vi "Start.vi"() -> ()   [LabVIEW 2017]
uses:
  <vilib>/Utility/config.llb/NI_LVConfig.lvlib
panel:
  out "Automation":bool
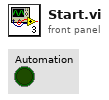
[diagram p1: front panel]
types:
  T1 = enum16{"End", "Start", "Verify VR", "Verify UUT"}
  T2 = enum16{"Auxiliary", "Temp Sens Cal", "Com Test", "Enable Test", "Speed Command", "Stop Time", "Temp Control", "Burn in", "Visual Inspec", "Empty"}
  T3 = enum16{"Auxiliary", "Temp Sens Cal", "Com Test", "Enable Test", "Speed Command", "Stop Time", "Temp Control", "Burn in", "Visual Inspec", "Empty"}[]
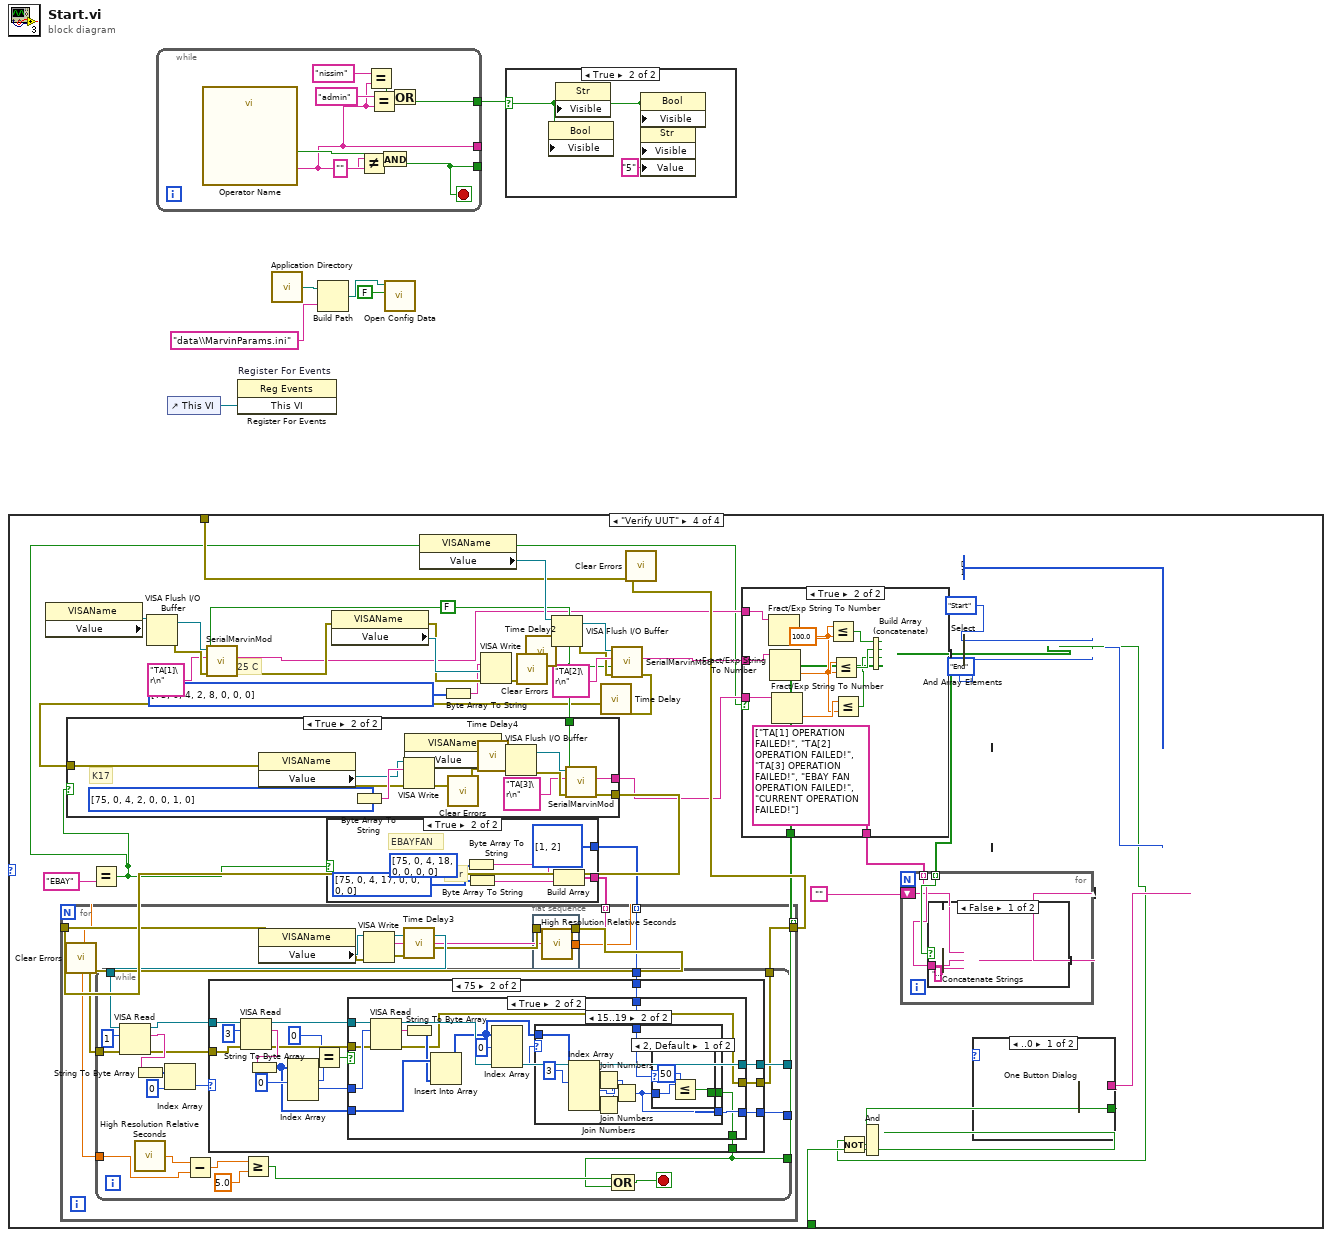
[diagram p0: block diagram]
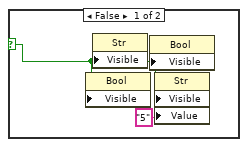
[diagram p2: hidden frame]
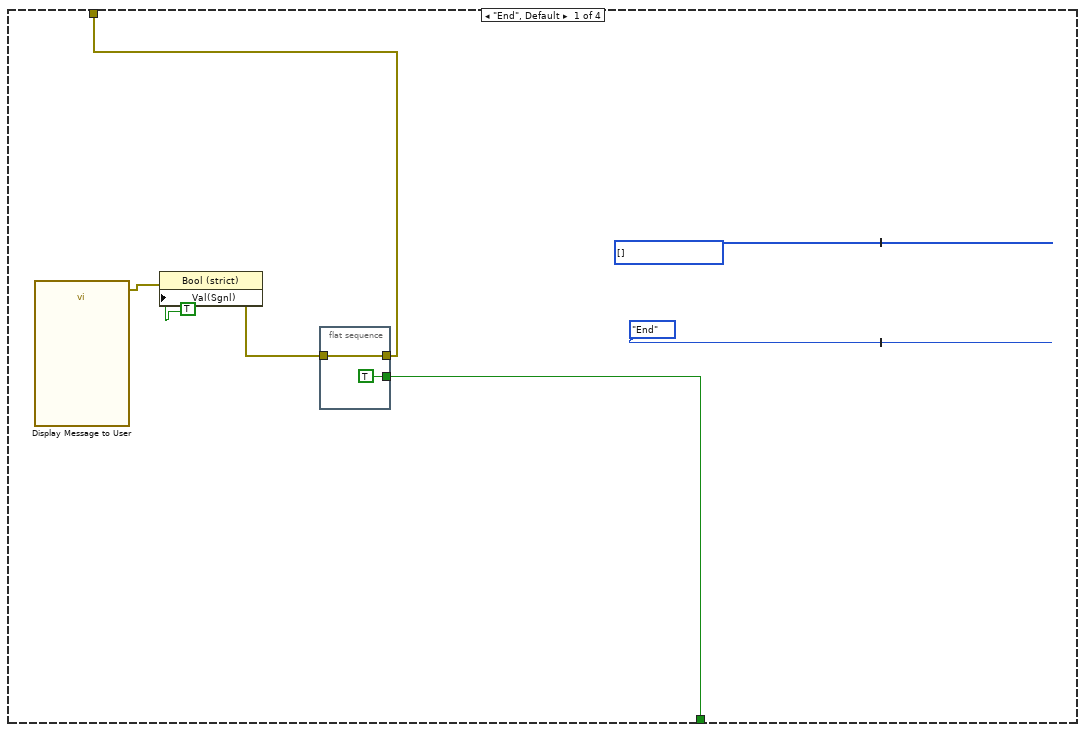
[diagram p3: hidden frame]
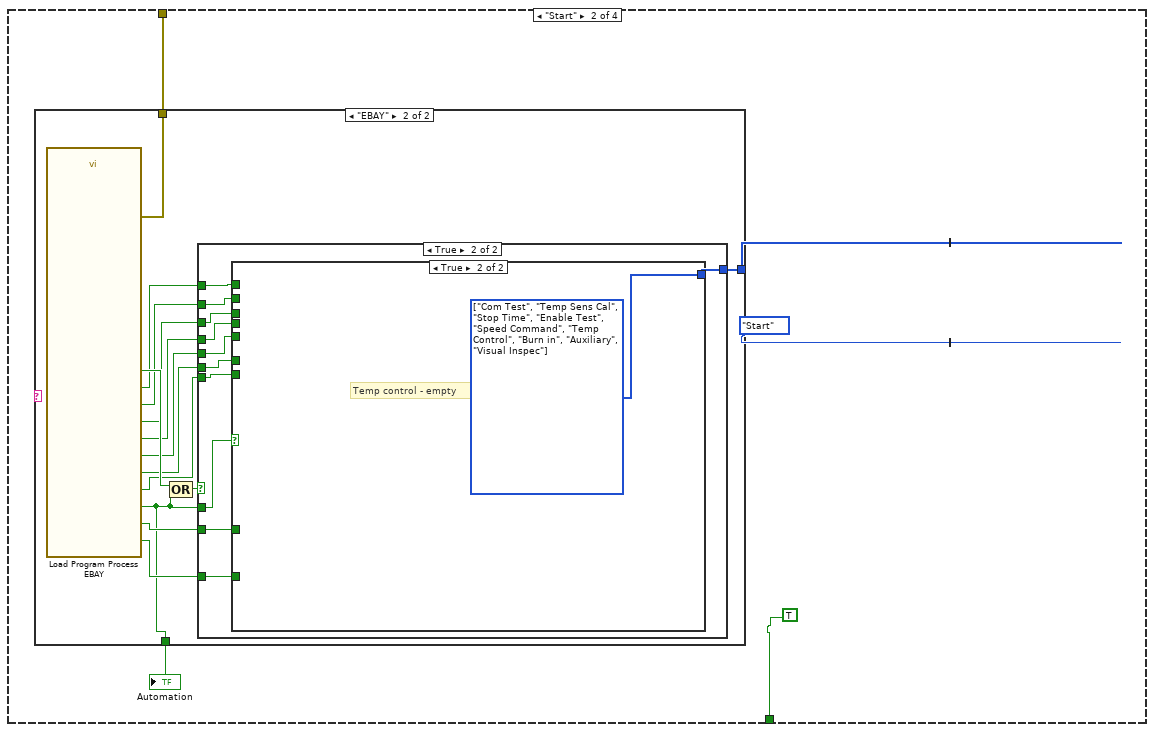
[diagram p4: hidden frame]
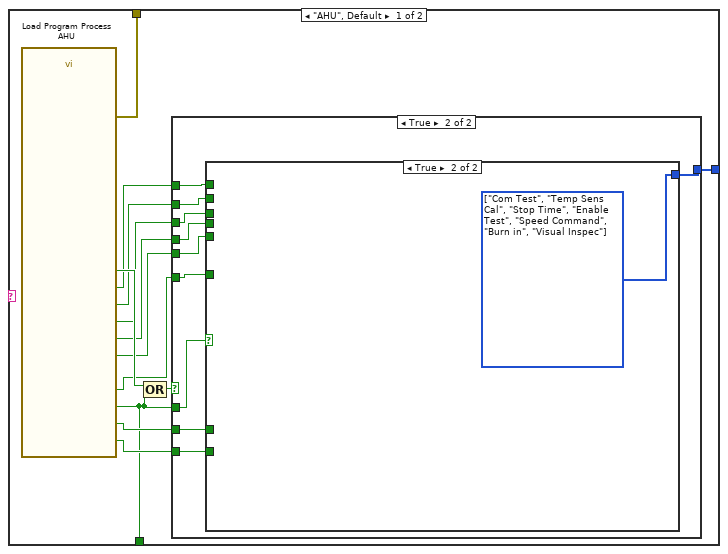
[diagram p5: hidden frame]
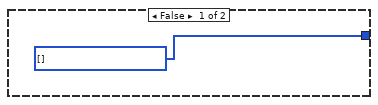
[diagram p6: hidden frame]
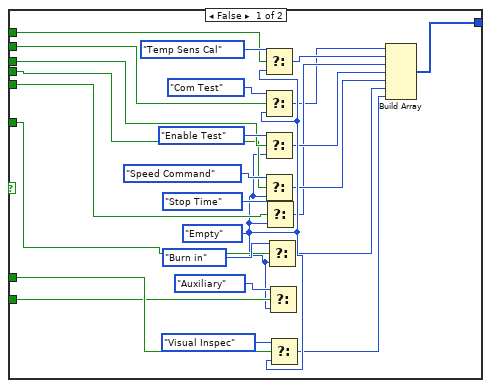
[diagram p7: hidden frame]
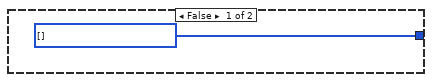
[diagram p8: hidden frame]
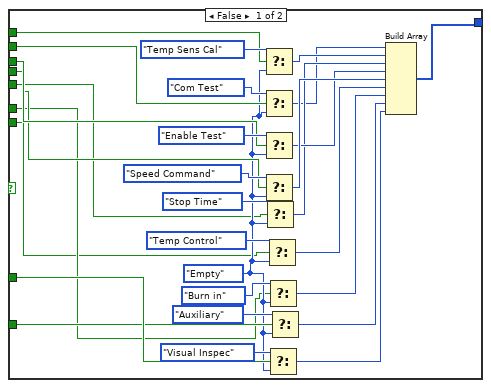
[diagram p9: hidden frame]
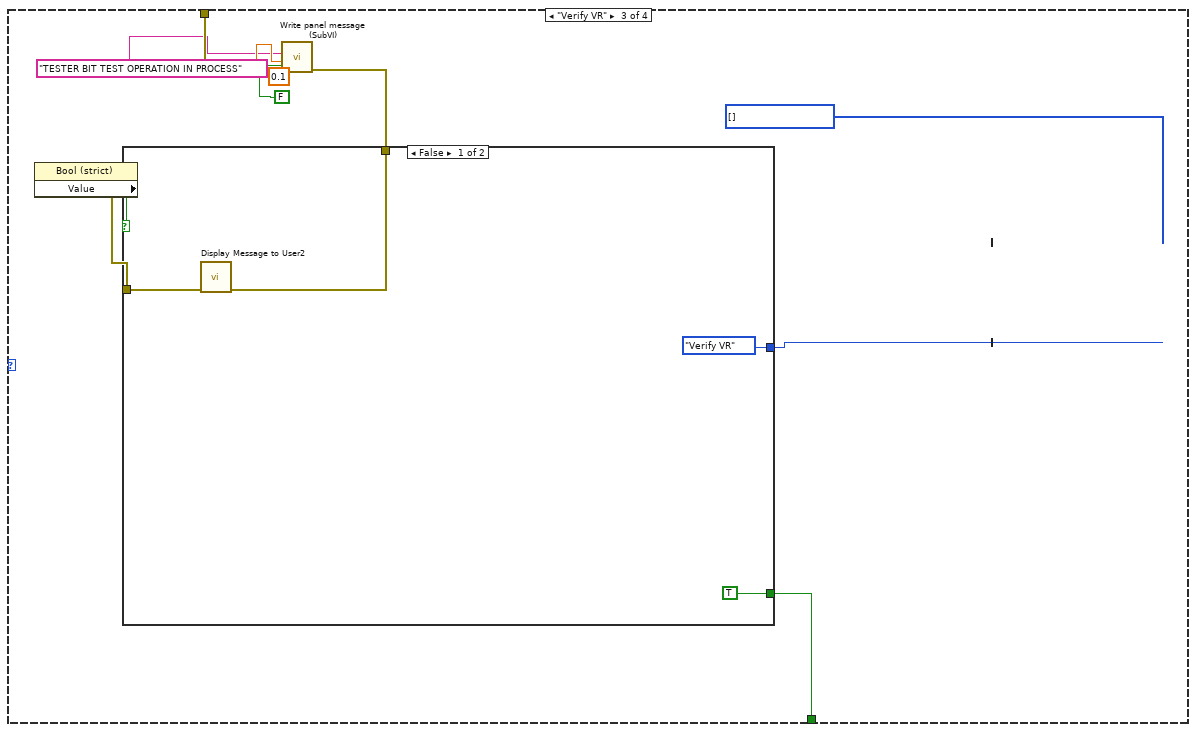
[diagram p10: hidden frame]
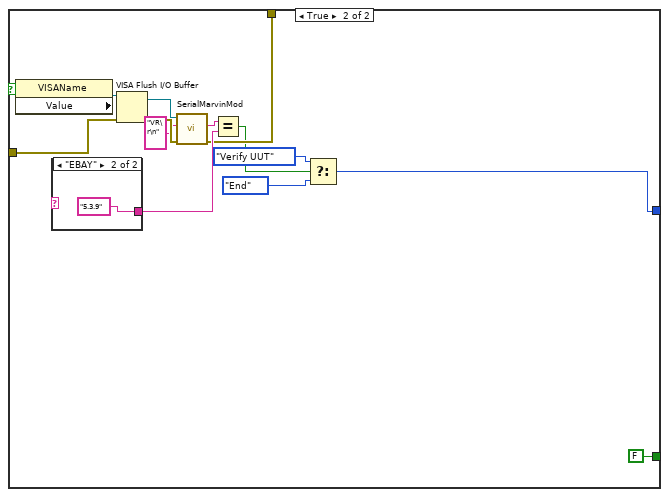
[diagram p11: hidden frame]
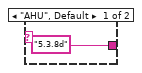
[diagram p12: hidden frame]
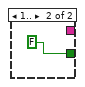
[diagram p13: hidden frame]
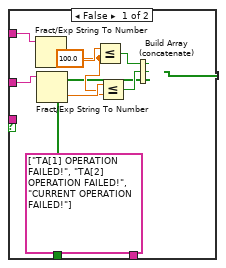
[diagram p14: hidden frame]
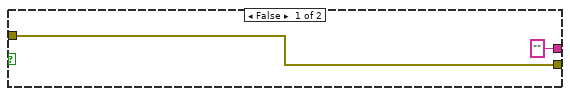
[diagram p15: hidden frame]
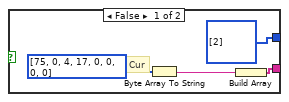
[diagram p16: hidden frame]
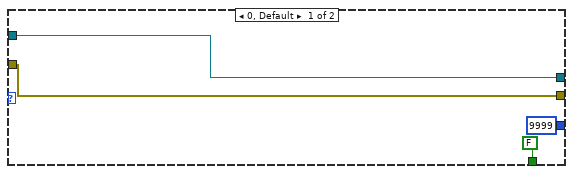
[diagram p17: hidden frame]
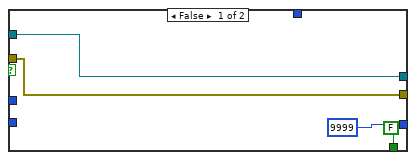
[diagram p18: hidden frame]
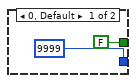
[diagram p19: hidden frame]
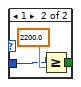
[diagram p20: hidden frame]
diagram:
  n1 = case shown="\"Verify UUT\"" {
    selector: _ -> [_ _ _ _]
    tunnel: [w10 w20 w130 w178] -> _
    tunnel: [w12 w19 w135 w156] -> _
    tunnel: [T1."End" T1."Start" w136 w172] -> _
    tunnel: [w11 TRUE w131 w166] -> _
    frame "End", Default {
      w12 = T3 [] items=["Auxiliary", "Temp Sens Cal", "Com Test", "Enable Test", "Speed Command", "Stop Time", "Temp Control", "Burn in", "Visual Inspec", "Empty"]
      n2 = call "Display Message to User"() -> ("error out"=w7:errorcluster)  [unwired: 10 in, 1 out]
      n3 = property on="Property Node" class="Bool (strict)"(error in=w7, "Val(Sgnl)"=TRUE ("Value (Signaling)")) -> (error out=w8:errorcluster)  [unwired: 1 in, 1 out]
      n4 = flat-sequence {
        tunnel: w8 -> [w14]
        tunnel: [TRUE] -> w11
        tunnel: [w14] -> w10
        frame #0 {
        }
      }
    }
    frame "Start" {
      n5 = case shown="\"EBAY\"" {
        selector: _ -> [_ _]
        tunnel: [w33 w84] -> w19
        tunnel: [w32 w83] -> w20
        tunnel: [w21 w71] -> w16
        frame "AHU", Default {
          n6 = call "Load Program Process AHU.vi"() -> ("Speed Command Test"=w26:bool, "Enable Test"=w27:bool, "Burn-in Test"=w24:bool, "Auxiliary"=w22:bool, "Temperature Sensor Calibration Test"=w29:bool, "Communication Test"=w28:bool, "Motor Temperature Test"=w25:bool, "Visual Inspection"=w23:bool, "OK"=w30:bool, "Automation"=w21:bool, "error out"=w32:errorcluster)  [unwired: 8 in, 9 out]
          n7 = Compound Arithmetic op=OR(w30, w21) -> (w31:bool)
          n8 = case shown="True" w31 {
            tunnel: [w34 w44] -> w33
            tunnel: w21 -> [_ w43]
            tunnel: w29 -> [_ w42]
            tunnel: w28 -> [_ w41]
            tunnel: w27 -> [_ w40]
            tunnel: w26 -> [_ w39]
            tunnel: w25 -> [_ w38]
            tunnel: w24 -> [_ w37]
            tunnel: w23 -> [_ w36]
            tunnel: w22 -> [_ w35]
            frame False {
              w34 = T3 [] items=["Auxiliary", "Temp Sens Cal", "Com Test", "Enable Test", "Speed Command", "Stop Time", "Temp Control", "Burn in", "Visual Inspec", "Empty"]
            }
            frame True {
              n9 = case shown="True" w43 {
                tunnel: [w69 w70] -> w44
                tunnel: w42 -> [w61 _]
                tunnel: w41 -> [w60 _]
                tunnel: w40 -> [w59 _]
                tunnel: w39 -> [w58 _]
                tunnel: w38 -> [w57 _]
                tunnel: w37 -> [w56 _]
                tunnel: w36 -> [w55 _]
                tunnel: w35 -> [w54 _]
                frame False {
                  w52 = T2."Empty" ("f")
                  n10 = Select(t=T2."Temp Sens Cal" ("f"), s=w61, f=w52) -> (s? t:f=w46:T2)
                  n11 = Select(t=T2."Com Test" ("f"), s=w60, f=w52) -> (s? t:f=w45:T2)
                  n12 = Select(t=T2."Enable Test" ("f"), s=w59, f=w52) -> (s? t:f=w48:T2)
                  n13 = Select(t=T2."Speed Command" ("f"), s=w58, f=w52) -> (s? t:f=w49:T2)
                  n14 = Select(t=T2."Stop Time" ("f"), s=w57, f=w52) -> (s? t:f=w47:T2)
                  n15 = Select(t=T2."Burn in" ("f"), s=w56, f=w52) -> (s? t:f=w50:T2)
                  n16 = Select(t=T2."Auxiliary" ("f"), s=w54, f=w52) -> ()  [unwired: 1 out]
                  n17 = Select(t=T2."Visual Inspec" ("f"), s=w55, f=w52) -> (s? t:f=w51:T2)
                  n18 = Build Array(w45, w46, w47, w48, w49, w50, w51) -> (w69:T3)
                }
                frame True {
                  w70 = T3 [enum."Com Test", enum."Temp Sens Cal", enum."Stop Time", enum."Enable Test", enum."Speed Command", enum."Burn in", enum."Visual Inspec"] items=["Auxiliary", "Temp Sens Cal", "Com Test", "Enable Test", "Speed Command", "Stop Time", "Temp Control", "Burn in", "Visual Inspec", "Empty"]
                }
              }
            }
          }
        }
        frame "EBAY" {
          n19 = call "Load Program Process EBAY.vi"() -> ("Speed Command Test"=w77:bool, "Enable Test"=w78:bool, "Burn-in Test"=w75:bool, "Temperature Control Algorithm Test"=w74:bool, "Auxiliary"=w72:bool, "Temperature Sensor Calibration Test"=w80:bool, "Communication Test"=w79:bool, "Motor Temperature Test"=w76:bool, "Visual Inspection"=w73:bool, "OK"=w81:bool, "Automation"=w71:bool, "error out"=w83:errorcluster)  [unwired: 8 in, 8 out]
          n20 = Compound Arithmetic op=OR(w81, w71) -> (w82:bool)
          n21 = case shown="True" w82 {
            tunnel: [w85 w96] -> w84
            tunnel: w71 -> [_ w95]
            tunnel: w80 -> [_ w94]
            tunnel: w79 -> [_ w93]
            tunnel: w78 -> [_ w92]
            tunnel: w77 -> [_ w91]
            tunnel: w76 -> [_ w90]
            tunnel: w75 -> [_ w89]
            tunnel: w74 -> [_ w88]
            tunnel: w73 -> [_ w87]
            tunnel: w72 -> [_ w86]
            frame False {
              w85 = T3 [] items=["Auxiliary", "Temp Sens Cal", "Com Test", "Enable Test", "Speed Command", "Stop Time", "Temp Control", "Burn in", "Visual Inspec", "Empty"]
            }
            frame True {
              n22 = case shown="True" w95 {
                tunnel: [w125 w126] -> w96
                tunnel: w94 -> [w116 _]
                tunnel: w93 -> [w115 _]
                tunnel: w92 -> [w114 _]
                tunnel: w91 -> [w113 _]
                tunnel: w90 -> [w103 _]
                tunnel: w89 -> [w108 _]
                tunnel: w88 -> [w107 _]
                tunnel: w87 -> [w112 _]
                tunnel: w86 -> [w111 _]
                frame False {
                  w109 = T2."Empty" ("f")
                  n23 = Select(t=T2."Temp Sens Cal" ("f"), s=w116, f=w109) -> (s? t:f=w98:T2)
                  n24 = Select(t=T2."Com Test" ("f"), s=w115, f=w109) -> (s? t:f=w97:T2)
                  n25 = Select(t=T2."Enable Test" ("f"), s=w114, f=w109) -> (s? t:f=w100:T2)
                  n26 = Select(t=T2."Speed Command" ("f"), s=w113, f=w109) -> (s? t:f=w101:T2)
                  n27 = Select(t=T2."Stop Time" ("f"), s=w103, f=w109) -> (s? t:f=w99:T2)
                  n28 = Select(t=T2."Temp Control" ("f"), s=w107, f=w109) -> (s? t:f=w102:T2)
                  n29 = Select(t=T2."Burn in" ("f"), s=w108, f=w109) -> (s? t:f=w104:T2)
                  n30 = Select(t=T2."Visual Inspec" ("f"), s=w112, f=w109) -> (s? t:f=w106:T2)
                  n31 = Select(t=T2."Auxiliary" ("f"), s=w111, f=w109) -> (s? t:f=w105:T2)
                  n32 = Build Array(w97, w98, w99, w100, w101, w102, w104, w105, w106) -> (w125:T3)
                }
                frame True {
                  w126 = T3 [enum."Com Test", enum."Temp Sens Cal", enum."Stop Time", enum."Enable Test", enum."Speed Command", enum."Temp Control", enum."Burn in", enum."Auxiliary", enum."Visual Inspec"] items=["Auxiliary", "Temp Sens Cal", "Com Test", "Enable Test", "Speed Command", "Stop Time", "Temp Control", "Burn in", "Visual Inspec", "Empty"]
                  # "Temp control - empty"
                }
              }
            }
          }
        }
      }
      "Automation" <- w16
    }
    frame "Verify VR" {
      w135 = T3 [] items=["Auxiliary", "Temp Sens Cal", "Com Test", "Enable Test", "Speed Command", "Stop Time", "Temp Control", "Burn in", "Visual Inspec", "Empty"]
      n33 = property on="Property Node" class="Bool (strict)"() -> (error out=w133:errorcluster, "Value"=w132:bool)  [unwired: 2 in, 1 out]
      n34 = case shown="False" w132 {
        tunnel: w133 -> [w140 w149]
        tunnel: [T1."Verify VR" w144] -> w136
        tunnel: [w138 w143] -> w134
        tunnel: [TRUE FALSE] -> w131
        frame False {
          n35 = call "Display Message to User2"("error in (no error)"=w140) -> ("error out"=w138:errorcluster)  [unwired: 9 in, 1 out]
        }
        frame True {
          n36 = property on="Property Node" class="VISAName"() -> ("Value"=w151:refnum<visa-resource-name>)  [unwired: 2 in, 2 out]
          n37 = case shown="\"EBAY\"" {
            selector: _ -> [_ _]
            tunnel: ["5.3.8d" ("write buffer") "5.3.9" ("write buffer")] -> w147
            frame "AHU", Default {
            }
            frame "EBAY" {
            }
          }
          n38 = VISA Flush I/O Buffer(VISA resource name=w151, error in (no error)=w149) -> (VISA resource name out=w153:refnum<visa-resource-name>, error out=w152:errorcluster)  [unwired: 1 in]
          n39 = call "SerialMarvinMod.vi"("error in (no error)"=w152, "write buffer"="VR\r\n", "VISA resource name"=w153) -> ("error out"=w143:errorcluster, "read buffer"=w148:string)  [unwired: 7 in]
          n40 = Equal?(x=w148, y=w147) -> (x = y?=w142:bool)
          n41 = Select(t=T1."Verify UUT", s=w142, f=T1."End") -> (s? t:f=w144:T1)
        }
      }
      n42 = call "Write panel message (SubVI).vi"("PrintTime"=FALSE, "error in (no error)"=w134, "Time to wait"=0.1, "Strin"="TESTER BIT TEST OPERATION IN PROCESS") -> ("error out"=w130:errorcluster)  [unwired: 7 in]
    }
    frame "Verify UUT" {
      w181 = FALSE ("Clear Log")
      w156 = T3 [] items=["Auxiliary", "Temp Sens Cal", "Com Test", "Enable Test", "Speed Command", "Stop Time", "Temp Control", "Burn in", "Visual Inspec", "Empty"]
      # "25 C"
      n43 = property on="Property Node" class="VISAName"() -> ("Value"=w195:refnum<visa-resource-name>)  [unwired: 2 in, 2 out]
      n44 = Equal?(y="EBAY") -> (x = y?=w158:bool)  [unwired: 1 in]
      n45 = VISA Flush I/O Buffer(VISA resource name=w195) -> (VISA resource name out=w197:refnum<visa-resource-name>, error out=w196:errorcluster)  [unwired: 2 in]
      n46 = call "SerialMarvinMod.vi"("error in (no error)"=w196, "Clear Log"=w181, "write buffer"="TA[1]\r\n", "VISA resource name"=w197) -> ("error out"=w183:errorcluster, "read buffer"=w177:string)  [unwired: 6 in]
      n47 = case shown="True" w158 {
        tunnel: [w242 w246] -> w160
        tunnel: [i32[] [2] i32[] [1, 2]] -> w157
        frame False {
          # "Cur"
          n48 = Byte Array To String(unsigned byte array=u8[] [75, 0, 4, 17, 0, 0, 0, 0] ("appended array")) -> (string=w243:string)
          n49 = Build Array(w243) -> (w242:string[])
        }
        frame True {
          # "Cur"
          # "EBAYFAN"
          n50 = Byte Array To String(unsigned byte array=u8[] [75, 0, 4, 18, 0, 0, 0, 0] ("appended array")) -> (string=w247:string)
          n51 = Byte Array To String(unsigned byte array=u8[] [75, 0, 4, 17, 0, 0, 0, 0] ("appended array")) -> (string=w248:string)
          n52 = Build Array(w247, w248) -> (w246:string[])
        }
      }
      n53 = property class="VISAName"(error in=w183) -> (error out=w192:errorcluster, "Value"=w193:refnum<visa-resource-name>)  [unwired: 1 in, 1 out]
      n54 = property on="Property Node" class="VISAName"() -> ("Value"=w188:refnum<visa-resource-name>)  [unwired: 2 in, 2 out]
      n55 = Byte Array To String(unsigned byte array=u8[] [75, 0, 4, 2, 8, 0, 0, 0] ("appended array")) -> (string=w190:string)
      n56 = VISA Write(VISA resource name=w193, write buffer=w190, error in (no error)=w192) -> (error out=w185:errorcluster)  [unwired: 2 out]
      n57 = call <vilib>:"Clear Errors.vi"("error in (no error)"=w185) -> ("error out"=w184:errorcluster)  [unwired: 5 in, 1 out]
      n58 = call "Time Delay2"("error in (no error)"=w184) -> ("error out"=w162:errorcluster)  [unwired: 10 in]
      n59 = VISA Flush I/O Buffer(VISA resource name=w188, error in (no error)=w162) -> (VISA resource name out=w186:refnum<visa-resource-name>, error out=w187:errorcluster)  [unwired: 1 in]
      n60 = call "SerialMarvinMod.vi"("error in (no error)"=w187, "Clear Log"=w181, "write buffer"="TA[2]\r\n", "VISA resource name"=w186) -> ("error out"=w182:errorcluster, "read buffer"=w176:string)  [unwired: 6 in]
      n61 = call "Time Delay"("error in (no error)"=w182) -> ("error out"=w163:errorcluster)  [unwired: 10 in]
      n62 = case shown="True" w158 {
        tunnel: w181 -> [_ w230]
        tunnel: [w224 w229] -> w180
        tunnel: ["" ("read buffer") w228] -> w175
        tunnel: w163 -> [w224 w227]
        frame False {
        }
        frame True {
          # "K17"
          n63 = property class="VISAName"(error in=w227) -> (error out=w238:errorcluster, "Value"=w237:refnum<visa-resource-name>)  [unwired: 1 in, 1 out]
          n64 = Byte Array To String(unsigned byte array=u8[] [75, 0, 4, 2, 0, 0, 1, 0] ("appended array")) -> (string=w240:string)
          n65 = VISA Write(VISA resource name=w237, write buffer=w240, error in (no error)=w238) -> (error out=w232:errorcluster)  [unwired: 2 out]
          n66 = property on="Property Node" class="VISAName"() -> ("Value"=w234:refnum<visa-resource-name>)  [unwired: 2 in, 2 out]
          n67 = call <vilib>:"Clear Errors.vi"("error in (no error)"=w232) -> ("error out"=w231:errorcluster)  [unwired: 5 in, 1 out]
          n68 = call "Time Delay4"("error in (no error)"=w231) -> ("error out"=w226:errorcluster)  [unwired: 10 in]
          n69 = VISA Flush I/O Buffer(VISA resource name=w234, error in (no error)=w226) -> (VISA resource name out=w236:refnum<visa-resource-name>, error out=w235:errorcluster)  [unwired: 1 in]
          n70 = call "SerialMarvinMod.vi"("error in (no error)"=w235, "Clear Log"=w230, "write buffer"="TA[3]\r\n", "VISA resource name"=w236) -> ("error out"=w229:errorcluster, "read buffer"=w228:string)  [unwired: 6 in]
        }
      }
      n71 = for {
        tunnel: [w254] -> w174 mode=indexing
        tunnel: w160 -> [w252] mode=indexing
        tunnel: w180 -> [w261]
        tunnel: [w255] -> w179
        tunnel: w157 -> [w251] mode=indexing
        n72 = call <vilib>:"Clear Errors.vi"("error in (no error)"=w257) -> ("error out"=w259:errorcluster)  [unwired: 5 in, 1 out]
        n73 = property class="VISAName"(error in=w261) -> (error out=w262:errorcluster, "Value"=w263:refnum<visa-resource-name>)  [unwired: 1 in, 1 out]
        n74 = VISA Write(VISA resource name=w263, write buffer=w252, error in (no error)=w262) -> (VISA resource name out=w260:refnum<visa-resource-name>, error out=w258:errorcluster)  [unwired: 1 out]
        n75 = while {
          tunnel: w259 -> [w278]
          tunnel: [w277] -> _
          tunnel: w256 -> [w275]
          tunnel: [w270] -> _
          tunnel: w260 -> [w269]
          tunnel: [w268] -> w255
          tunnel: [w267] -> w254
          tunnel: w251 -> [w266]
          stop <- w271 stop-if-true
          n76 = VISA Read(VISA resource name=w269, byte count=u32 1, error in (no error)=w278) -> (VISA resource name out=w280:refnum<visa-resource-name>, read buffer=w281:string, error out=w279:errorcluster)  [unwired: 1 out]
          n77 = String To Byte Array(string=w281) -> (unsigned byte array=w284:u8[])
          n78 = call <vilib>:"High Resolution Relative Seconds.vi"() -> ("relative seconds"=w276:dbl)
          n79 = Index Array(array=w284, index=0) -> (element=w282:u8)
          n80 = Subtract(x=w276, y=w275) -> (x-y=w274:dbl)
          n81 = case shown="75" w282 {
            tunnel: [w289 w294] -> w268
            tunnel: w280 -> [w288 w303]
            tunnel: w279 -> [w289 w302]
            tunnel: [w288 w295] -> w277
            tunnel: [u32 9999 w292] -> w270
            tunnel: [FALSE w291] -> w267
            tunnel: w266 -> [_ w290]
            frame 0, Default {
            }
            frame 75 {
              n82 = VISA Read(VISA resource name=w303, byte count=u32 3, error in (no error)=w302) -> (VISA resource name out=w298:refnum<visa-resource-name>, read buffer=w306:string, error out=w297:errorcluster)  [unwired: 1 out]
              n83 = String To Byte Array(string=w306) -> (unsigned byte array=w296:u8[])
              n84 = Index Array(array=w296, index #1=0 ("index")) -> (element #1=w301:u8, element #2=w299:u8)  [unwired: 2 in, 1 out]
              n85 = Equal?(x=u8 0, y=w301) -> (x = y?=w300:bool)
              n86 = case shown="True" w300 {
                tunnel: [w309 w317] -> w294
                tunnel: w299 -> [_ w324]
                tunnel: w298 -> [w310 w323]
                tunnel: w297 -> [w309 w322]
                tunnel: w296 -> [_ w321]
                tunnel: [w310 w319] -> w295
                tunnel: [u32 9999 w313] -> w292
                tunnel: [FALSE w312] -> w291
                tunnel: w290 -> [_ w311]
                frame False {
                }
                frame True {
                  n87 = VISA Read(VISA resource name=w323, byte count=w324, error in (no error)=w322) -> (VISA resource name out=w319:refnum<visa-resource-name>, read buffer=w318:string, error out=w317:errorcluster)  [unwired: 1 out]
                  n88 = String To Byte Array(string=w318) -> (unsigned byte array=w320:u8[])
                  n89 = Insert Into Array(array=w321, new element=w320) -> (w314:u8[])  [unwired: 1 in]
                  n90 = Index Array(array=w314, index #1=0 ("index")) -> (element #3=w315:u8)  [unwired: 2 in, 2 out]
                  n91 = case shown="15..19" w315 {
                    tunnel: w314 -> [_ w336]
                    tunnel: [u32 9999 w328] -> w313
                    tunnel: [FALSE w329] -> w312
                    tunnel: w311 -> [_ w327]
                    frame 0, Default {
                    }
                    frame 15..19 {
                      n92 = Index Array(array=w336, index #1=3 ("index")) -> (element #1=w335:u8, element #2=w334:u8, element #3=w333:u8, element #4=w332:u8)  [unwired: 3 in]
                      n93 = Join Numbers(hi=w334, lo=w335) -> ((hi.lo)=w331:u16)
                      n94 = Join Numbers(hi=w332, lo=w333) -> ((hi.lo)=w330:u16)
                      n95 = Join Numbers(hi=w330, lo=w331) -> ((hi.lo)=w328:u32)
                      n96 = case shown="2, Default" w327 {
                        tunnel: [w338 w342] -> w329
                        tunnel: w328 -> [w340 w341]
                        frame 2, Default {
                          n97 = Less Or Equal?(x=w340, y=u32 50) -> (x <= y?=w338:bool)
                        }
                        frame 1 {
                          n98 = Greater Or Equal?(x=w341, y=2200.0) -> (x >= y?=w342:bool)
                        }
                      }
                    }
                  }
                }
              }
            }
          }
          n99 = Greater Or Equal?(x=w274, y=5.0) -> (x >= y?=w272:bool)
          n100 = Compound Arithmetic op=OR(w272, w267) -> (w271:bool)
        }
        n101 = call "Time Delay3"("error in (no error)"=w258) -> ("error out"=w253:errorcluster)  [unwired: 10 in]
        n102 = flat-sequence {
          tunnel: w253 -> [w265]
          tunnel: [w265] -> w257
          tunnel: [w264] -> w256
          frame #0 {
            n103 = call <vilib>:"High Resolution Relative Seconds.vi"() -> ("relative seconds"=w264:dbl)
          }
        }
      }
      n104 = call <vilib>:"Clear Errors.vi"("error in (no error)"=w179) -> ("error out"=w178:errorcluster)  [unwired: 5 in, 1 out]
      n105 = case shown="True" w158 {
        tunnel: w177 -> [w210 w223]
        tunnel: w176 -> [w209 w222]
        tunnel: w175 -> [_ w221]
        tunnel: w174 -> [w203 w213]
        tunnel: [w202 w212] -> w170
        tunnel: [string[] ["TA[1] OPERATION FAILED!", "TA[2] OPERATION FAILED!", "CURRENT OPERATION FAILED!"] string[] ["TA[1] OPERATION FAILED!", "TA[2] OPERATION FAILED!", "TA[3] OPERATION FAILED!", "EBAY FAN OPERATION FAILED!", "CURRENT OPERATION FAILED!"]] -> w169
        frame False {
          w206 = 100.0 ("y")
          n106 = Fract/Exp String To Number(string=w210) -> (number=w208:dbl)  [unwired: 3 in, 1 out]
          n107 = Fract/Exp String To Number(string=w209) -> (number=w207:dbl)  [unwired: 3 in, 1 out]
          n108 = Less Or Equal?(x=w208, y=w206) -> (x <= y?=w205:bool)
          n109 = Less Or Equal?(x=w207, y=w206) -> (x <= y?=w204:bool)
          n110 = Build Array (concatenate)(w205, w204, w203) -> (w202:bool[])
        }
        frame True {
          w217 = 100.0 ("y")
          n111 = Fract/Exp String To Number(string=w223) -> (number=w220:dbl)  [unwired: 3 in, 1 out]
          n112 = Fract/Exp String To Number(string=w222) -> (number=w219:dbl)  [unwired: 3 in, 1 out]
          n113 = Fract/Exp String To Number(string=w221) -> (number=w218:dbl)  [unwired: 3 in, 1 out]
          n114 = Less Or Equal?(x=w220, y=w217) -> (x <= y?=w216:bool)
          n115 = Less Or Equal?(x=w219, y=w217) -> (x <= y?=w215:bool)
          n116 = Less Or Equal?(x=w218, y=w217) -> (x <= y?=w214:bool)
          n117 = Build Array (concatenate)(w216, w215, w214, w213) -> (w212:bool[])
        }
      }
      n118 = for {
        tunnel: w170 -> [w347] mode=indexing
        tunnel: w169 -> [w346] mode=indexing
        shift-right: [w344] -> w167
        shift-left: "" -> [w345]
        n119 = case shown="False" w347 {
          tunnel: w346 -> [w350 _]
          tunnel: w345 -> [w351 w352]
          tunnel: [w348 w352] -> w344
          frame False {
            n120 = Concatenate Strings(w351, w350, "\r\n") -> (w348:string)
          }
          frame True {
          }
        }
      }
      n121 = And Array Elements(Boolean array=w170) -> (logical AND=w161:bool)
      n122 = Not(x=w161) -> (.not. x?=w164:bool)
      n123 = Select(t=T1."Start", s=w161, f=T1."End") -> (s? t:f=w172:T1)
      n124 = case shown="..0" {
        tunnel: w167 -> [w199 _]
        tunnel: [w198 FALSE ("true")] -> w165
        selector: _ -> [_ _]
        frame ..0 {
          n125 = One Button Dialog(message=w199) -> (true=w198:bool)  [unwired: 1 in]
        }
        frame 1.. {
        }
      }
      n126 = And(x=w165, y=w164) -> (x .and. y?=w166:bool)
    }
  }
  n127 = while {
    tunnel: [w359] -> _
    tunnel: [w355] -> _
    tunnel: [w356] -> w1
    stop <- w359 stop-if-true
    n128 = call "Operator Name"() -> ("Operator Name"=w355:string, "OK"=w360:bool)  [unwired: 17 in, 1 out]
    n129 = Not Equal?(x=w355, y="") -> (x != y?=w361:bool)
    n130 = Equal?(x="nissim", y=w355) -> (x = y?=w353:bool)
    n131 = Equal?(x="admin", y=w355) -> (x = y?=w357:bool)
    n132 = And(x=w360, y=w361) -> (x .and. y?=w359:bool)
    n133 = Or(x=w353, y=w357) -> (x .or. y?=w356:bool)
  }
  n134 = control-ref of="This VI"() -> (w2:refnum<vi>)
  n135 = register-events "Register For Events"(w2) -> ()  [unwired: 2 in, 2 out]
  n136 = call <vilib>:"Application Directory.vi"() -> ("Application Directory"=w6:path)
  n137 = Build Path(base path=w6, name or relative path="data\\MarvinParams.ini") -> (appended path=w3:path)
  n138 = call <vilib>:"Open Config Data.vi"("create file if necessary (T)"=FALSE, "configuration file path"=w3) -> ()  [unwired: 1 in, 9 out]
  n139 = case shown="True" w1 {
    selector: w1 -> [w364 w366]
    frame False {
      n140 = property on="Property Node" class="Bool"("Visible"=w364) -> ()  [unwired: 2 in, 2 out]
      n141 = property on="Property Node" class="Str"("Visible"=w364) -> ()  [unwired: 2 in, 2 out]
      n142 = property on="Property Node" class="Bool"("Visible"=w364) -> ()  [unwired: 2 in, 2 out]
      n143 = property on="Property Node" class="Str"("Visible"=w364, "Value"="5" ("Index")) -> ()  [unwired: 2 in, 2 out]
    }
    frame True {
      n144 = property on="Property Node" class="Bool"("Visible"=w366) -> ()  [unwired: 2 in, 2 out]
      n145 = property on="Property Node" class="Str"("Visible"=w366) -> ()  [unwired: 2 in, 2 out]
      n146 = property on="Property Node" class="Bool"("Visible"=w366) -> ()  [unwired: 2 in, 2 out]
      n147 = property on="Property Node" class="Str"("Visible"=w366, "Value"="5" ("Index")) -> ()  [unwired: 2 in, 2 out]
    }
  }
